vi "Add Hardware.vi"(8 "error in (no error)":errorcluster, 10 "Hardware.lvclass":refnum<class "Hardware.lvclass">, 11 "Controller in":refnum<class "Controller.lvclass">) -> (0 "error out":errorcluster, 3 "Controller out":refnum<class "Controller.lvclass">)   [LabVIEW 2015, in "Controller Actor.lvlib" / "Controller.lvclass"]
uses:
  Controller.lvclass
  Hardware/Hardware.lvclass
  <vilib>/ActorFramework/Actor/Actor.lvclass/Actor.ctl
  <vilib>/ActorFramework/Message Enqueuer/Message Enqueuer.lvclass/Message Enqueuer.ctl
  <vilib>/ActorFramework/Message Enqueuer/Init from Existing Queue.vi
  <vilib>/ActorFramework/Message Enqueuer/Message Enqueuer.lvclass
  Messages/Log Status/Log Status.lvclass
  <vilib>/ActorFramework/Actor/Actor.lvclass
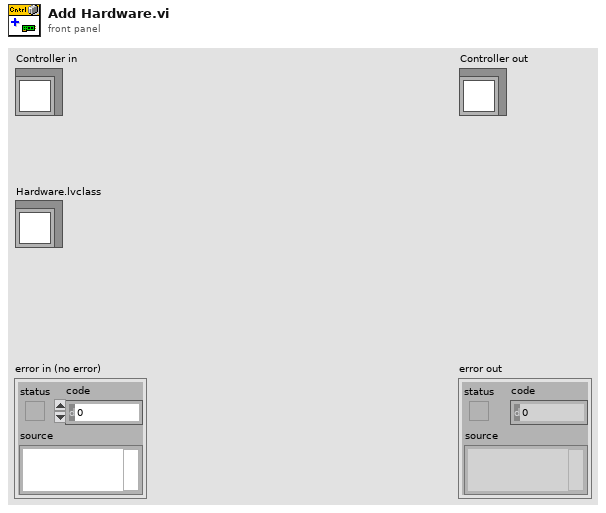
[diagram p1: front panel]
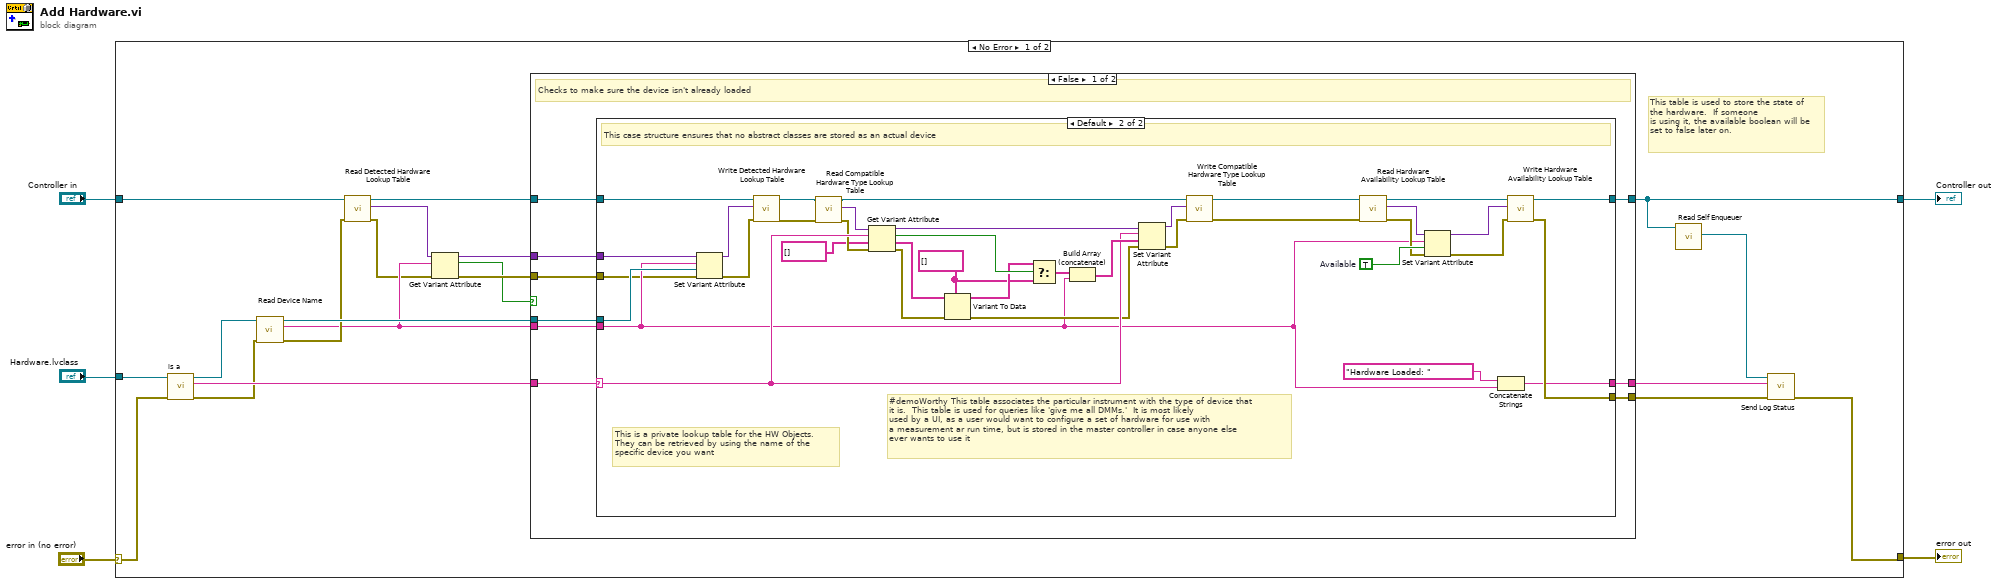
[diagram p0: block diagram]
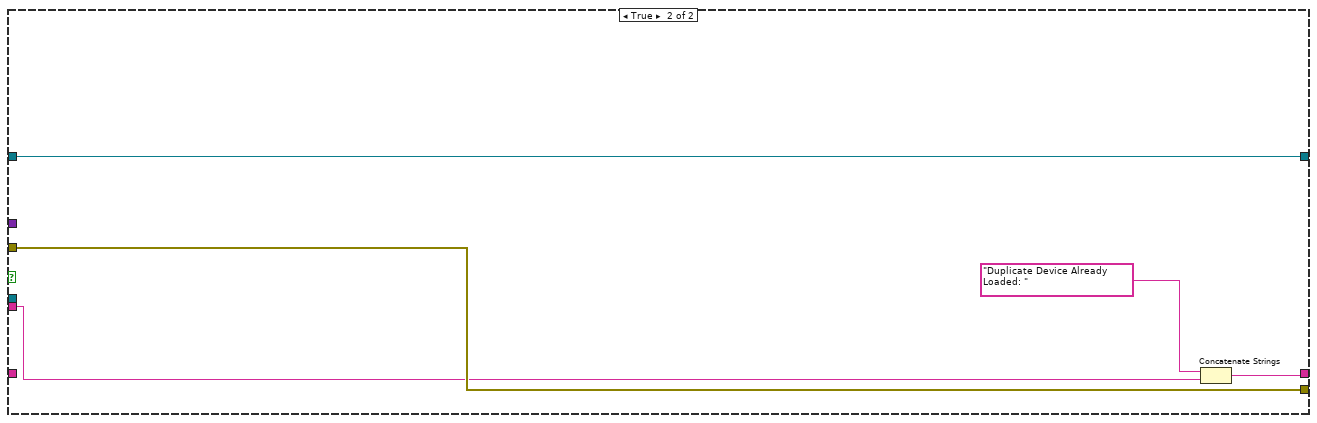
[diagram p3: hidden frame]
diagram:
  n1 = case shown="No Error" "error in (no error)" {
    selector: "error in (no error)" -> [w23 w79]
    tunnel: [w22 w79] -> w4
    tunnel: [w8 w78] -> w2
    tunnel: "Controller in" -> [w17 w78]
    tunnel: "Hardware.lvclass" -> [w20 _]
    frame No Error {
      # "This table is used to store the state of the hardware.  If someone\nis using it, the available boolean will be set to false later on."
      n2 = call-dynamic "is a.vi"("error in (no error)"=w23, "Hardware in"=w20) -> ("error out"=w18:errorcluster, "is a"=w24:string, "Hardware out"=w19:refnum<class "Hardware.lvclass">)  [unwired: 7 in]
      n3 = call "Read Device Name.vi"("error in (no error)"=w18, "Analog in"=w19) -> ("error out"=w15:errorcluster, "Device Name"=w12:string, "Analog out"=w21:refnum<class "Hardware.lvclass">)  [unwired: 7 in]
      n4 = call "Read Detected Hardware Lookup Table.vi"("error in (no error)"=w15, "Controller in"=w17) -> ("error out"=w11:errorcluster, "Detected Hardware Lookup Table"=w14:variant, "Controller out"=w16:refnum<class "Controller.lvclass">)  [unwired: 7 in]
      n5 = Get Variant Attribute(Variant=w14, name=w12, error in=w11) -> (duplicate Variant=w13:variant, found=w6:bool, error out=w10:errorcluster)  [unwired: 1 in, 1 out]
      n6 = case shown="False" w6 {
        tunnel: w24 -> [w33 _]
        tunnel: [w32 w76] -> w22
        tunnel: w21 -> [w31 _]
        tunnel: w16 -> [w30 w77]
        tunnel: w13 -> [w29 _]
        tunnel: w12 -> [w28 w73]
        tunnel: w10 -> [w27 w76]
        tunnel: [w26 w77] -> w8
        tunnel: [w25 w74] -> w7
        frame False {
          # "Checks to make sure the device isn't already loaded"
          n7 = case shown="Default" w33 {
            selector: w33 -> [_ w54]
            tunnel: w30 -> [w35 w40]
            tunnel: [w35 w55] -> w26
            tunnel: [w34 w37] -> w32
            tunnel: w31 -> [_ w42]
            tunnel: w28 -> [_ w41]
            tunnel: w29 -> [_ w39]
            tunnel: w27 -> [w34 w38]
            tunnel: [_ w36] -> w25
            frame "Abstract Class" {
            }
            frame Default {
              w60 = TRUE  # Available
              w66 = string[] []
              # "This is a private lookup table for the HW Objects.  \nThey can be retrieved by using the name of the\nspecific device you want"
              # "#demoWorthy This table associates the particular instrument with the type of device that\nit is.  This table is used for queries like 'give me all DMMs.'  It is most likely\nused by a UI, as a user would want to configure a set of hardware for use with\na measurement ar run time, but is stored in the master controller in case anyone else\never wants to use it"
              # "This case structure ensures that no abstract classes are stored as an actual device"
              n8 = Set Variant Attribute(Variant=w39, name=w41, value=w42, error in=w38) -> (Variant out=w72:variant, error out=w51:errorcluster)  [unwired: 1 out]
              n9 = call "Write Detected Hardware Lookup Table.vi"("error in (no error)"=w51, "Detected Hardware Lookup Table"=w72, "Controller in"=w40) -> ("error out"=w52:errorcluster, "Controller out"=w64:refnum<class "Controller.lvclass">)  [unwired: 7 in]
              n10 = call "Read Compatible Hardware Type Lookup Table.vi"("error in (no error)"=w52, "Controller in"=w64) -> ("error out"=w53:errorcluster, "Compatible Hardware Type Lookup Table"=w61:variant, "Controller out"=w63:refnum<class "Controller.lvclass">)  [unwired: 7 in]
              n11 = Get Variant Attribute(Variant=w61, name=w54, default value (empty Variant)=string[] [], error in=w53) -> (duplicate Variant=w65:variant, found=w69:bool, value=w71:string[], error out=w50:errorcluster)
              n12 = Variant To Data(error in=w50, type=w66, Variant=w71) -> (data=w67:string[], error out=w49:errorcluster)
              n13 = Select(t=w67, s=w69, f=w66) -> (s? t:f=w68:string[])
              n14 = Build Array (concatenate)(w68, w41) -> (w70:string[])
              n15 = Set Variant Attribute(Variant=w65, name=w54, value=w70, error in=w49) -> (Variant out=w62:variant, error out=w48:errorcluster)  [unwired: 1 out]
              n16 = call "Write Compatible Hardware Type Lookup Table.vi"("error in (no error)"=w48, "Compatible Hardware Type Lookup Table"=w62, "Controller in"=w63) -> ("error out"=w47:errorcluster, "Controller out"=w59:refnum<class "Controller.lvclass">)  [unwired: 7 in]
              n17 = call "Read Hardware Availability Lookup Table.vi"("error in (no error)"=w47, "Controller in"=w59) -> ("error out"=w46:errorcluster, "Hardware Availability Lookup Table"=w58:variant, "Controller out"=w56:refnum<class "Controller.lvclass">)  [unwired: 7 in]
              n18 = Set Variant Attribute(Variant=w58, name=w41, value=w60, error in=w46) -> (Variant out=w57:variant, error out=w45:errorcluster)  [unwired: 1 out]
              n19 = Concatenate Strings("Hardware Loaded: " ("string"), w41) -> (w36:string)
              n20 = call "Write Hardware Availability Lookup Table.vi"("error in (no error)"=w45, "Hardware Availability Lookup Table"=w57, "Controller in"=w56) -> ("error out"=w37:errorcluster, "Controller out"=w55:refnum<class "Controller.lvclass">)  [unwired: 7 in]
            }
          }
        }
        frame True {
          n21 = Concatenate Strings("Duplicate Device Already Loaded: " ("string"), w73) -> (w74:string)
        }
      }
      n22 = call <vilib>:"Read Self Enqueuer.vi"("Actor"=w8) -> ("Self Enqueuer"=w9:refnum<class "Message Enqueuer.lvclass">)  [unwired: 10 in]
      n23 = call "Send Log Status.vi"("String"=w7, "Message Enqueuer in"=w9) -> ()  [unwired: 8 in, 2 out]
    }
    frame Error {
    }
  }
  "error out" <- w4
  "Controller out" <- w2
